vi "changeLevel.vi"(8 "error in (no error)":errorcluster, 10 "Level":u8, 11 "Simon_Engine in":refnum<class "Simon_Engine.lvclass">) -> (0 "error out":errorcluster, 3 "Simon_Engine out":refnum<class "Simon_Engine.lvclass">)   [LabVIEW 2019, in "Simon_Engine.lvclass"]
uses:
  Simon_Engine.lvclass
  Simon_Engine.lvclass/Simon_Engine.ctl
  LED/LED Class/LED.lvclass
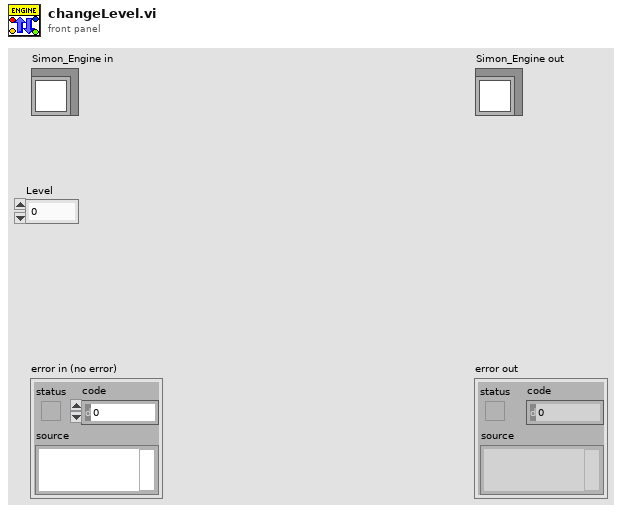
[diagram p1: front panel]
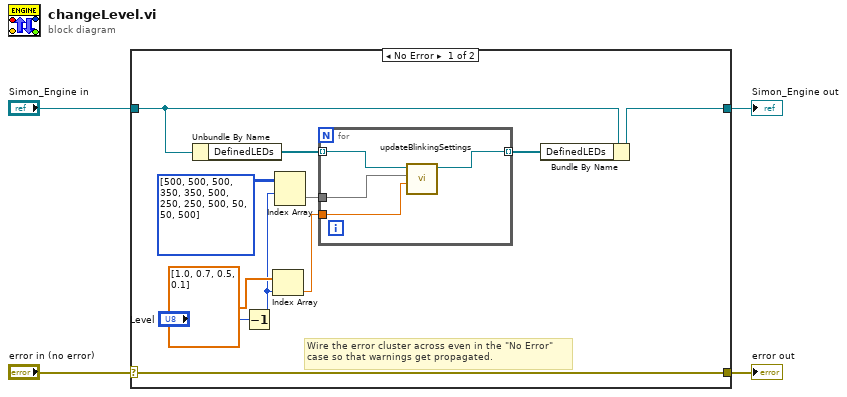
[diagram p0: block diagram]
diagram:
  n1 = case shown="No Error" "error in (no error)" {
    selector: "error in (no error)" -> [w15 w21]
    tunnel: [w15 w21] -> w3
    tunnel: [w10 w20] -> w1
    tunnel: "Simon_Engine in" -> [w14 w20]
    frame No Error {
      # "Wire the error cluster across even in the \"No Error\"\ncase so that warnings get propagated."
      n2 = Unbundle By Name(w14) -> ("DefinedLEDs"=w13:refnum<class "LED.lvclass">[])
      n3 = Decrement(x="Level") -> (x-1=w5:u8)
      n4 = Index Array(array=dbl[] [1.0, 0.7, 0.5, 0.1] ("Waveform Duration (s)"), index=w5) -> (element=w7:dbl)
      n5 = Index Array(array=u32[][] [[500, 500, 500], [350, 350, 500], [250, 250, 500], [50, 50, 500]] ("On and Off time (ms)"), index (row)=w5) -> (element=w12:u32[])  [unwired: 1 in]
      n6 = for {
        tunnel: w13 -> [w19] mode=indexing
        tunnel: w12 -> [w18]
        tunnel: [w17] -> w9 mode=indexing
        tunnel: w7 -> [w16]
        n7 = call "updateBlinkingSettings.vi"("Waveform Duration (s)"=w16, "On and Off time (ms)"=w18, "LED in"=w19) -> ("LED out"=w17:refnum<class "LED.lvclass">)  [unwired: 7 in, 1 out]
      }
      n8 = Bundle By Name(cluster=w14, "DefinedLEDs"=w9) -> (w10:refnum<class "Simon_Engine.lvclass">)
    }
    frame Error {
    }
  }
  "error out" <- w3
  "Simon_Engine out" <- w1
